vi "Read_CSV_To_Int_Array.vi"() -> ()   [LabVIEW 2016]
uses:
  <vilib>/Utility/file.llb/Read Delimited Spreadsheet (I64).vi
panel:
  out "first row":u16[](array[numeric])
  out "all rows":i64[][](array[numeric])
  in  "file path (dialog if empty)":path
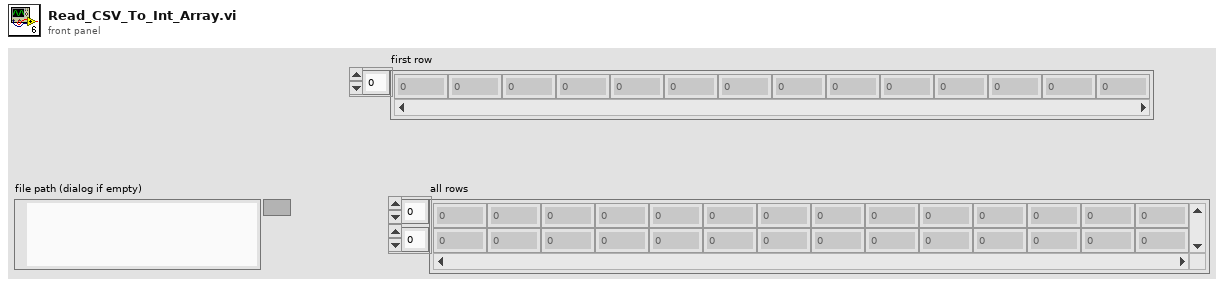
[diagram p1: front panel]
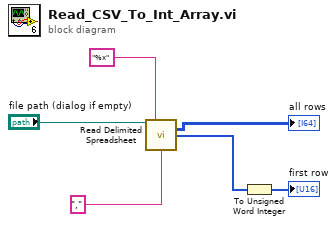
[diagram p0: block diagram]
diagram:
  n1 = call-poly <vilib>:"Read Delimited Spreadsheet.vi"("file path (dialog if empty)"="file path (dialog if empty)", "format (%d)"="%x", "delimiter (\\t)"="," ("delimiter (\\t)")) -> ("all rows"=→"all rows":i64[][], "first row"=w2:i64[])  [unwired: 7 in, 4 out]
  n2 = To Unsigned Word Integer(number=w2) -> (unsigned 16bit integer=→"first row":u16[])
